vi "Pack PII Error_1SDI_v00.vi"(8 "PII+Error HD C":T1, 9 "PII+Error HD B":T1, 10 "PII+Error HD A":T1, 11 "PII+Error EPR BS":T8) -> (0 "Theta":T5, 1 "Thresholds":cluster{"Lock":T7, "Re-Scan":T7}, 3 "Error packed":T6={"Pre-Offset"={"Pre-Offset 1"=2, "Pre-Offset 2"=0, "Pre-Offset 3"=0, "Pre-Offset 4"=0, "Pre-Offset 5"=2, "Pre-Offset 6"=0, "Pre-Offset 7"=2}, "Post-Offset "={"Offset 1"=0, "Offset 2"=0, "Offset 3"=0, "Offset 4"=0, "Offset 5"=0, "Offset 6"=0, "Offset 7"=0}, "Gains"={"Gain 1"=0, "Gain 2"=0, "Gain 3"=0, "Gain 4"=0, "Gain 5"=0, "Gain 6"=0, "Gain 7"=0}, "Bit Shifts"={"Bit Shift 1"=0, "Bit Shift 2"=300, "Bit Shift 3"=0, "Bit Shift 4"=0, "Bit Shift 5"=0, "Bit Shift 6"=0, "Bit Shift 7"=0}})   [LabVIEW 2013]
doc: "Packages individual values related to error signal scaling from the user interface into data structures compatible with FPGA_Cavities.VI\n(very messy, could use a tidy)."
uses:
  Strict Type Defs/1SDI Errors I16.ctl
  Strict Type Defs/Error Scale 1SDI.ctl
  Strict Type Defs/PII and Error Graph.ctl
  Strict Type Defs/Errors Converted Graph.ctl
  Strict Type Defs/PII individual.ctl
  Strict Type Defs/PII and Error Graph HD.ctl
  Strict Type Defs/Errors Converted Graph HD.ctl
  Strict Type Defs/Lock Thresh 1SDI.ctl
  Strict Type Defs/Theta graph.ctl
panel:
  in  "Bit Shifts":T4
  in  "Theta typedef":T5
  in  "Error scale graph type":T6={"Pre-Offset"={"Pre-Offset 1"=2, "Pre-Offset 2"=0, "Pre-Offset 3"=0, "Pre-Offset 4"=0, "Pre-Offset 5"=2, "Pre-Offset 6"=0, "Pre-Offset 7"=2}, "Post-Offset "={"Offset 1"=0, "Offset 2"=300, "Offset 3"=0, "Offset 4"=0, "Offset 5"=0, "Offset 6"=0, "Offset 7"=0}, "Gains"={"Gain 1"=0, "Gain 2"=300, "Gain 3"=0, "Gain 4"=0, "Gain 5"=0, "Gain 6"=0, "Gain 7"=0}, "Bit Shifts"={"Bit Shift 1"=0, "Bit Shift 2"=300, "Bit Shift 3"=0, "Bit Shift 4"=0, "Bit Shift 5"=0, "Bit Shift 6"=0, "Bit Shift 7"=0}}
  in  "Thresholds type def":cluster{"Lock":T7, "Re-Scan":T7}
  in  "Re-Scan Thresh":T7
  in  "Lock Thresh":T7
  in  "Pre Offset":T4
  in  "Offset":T4
  in  "Gains":T4
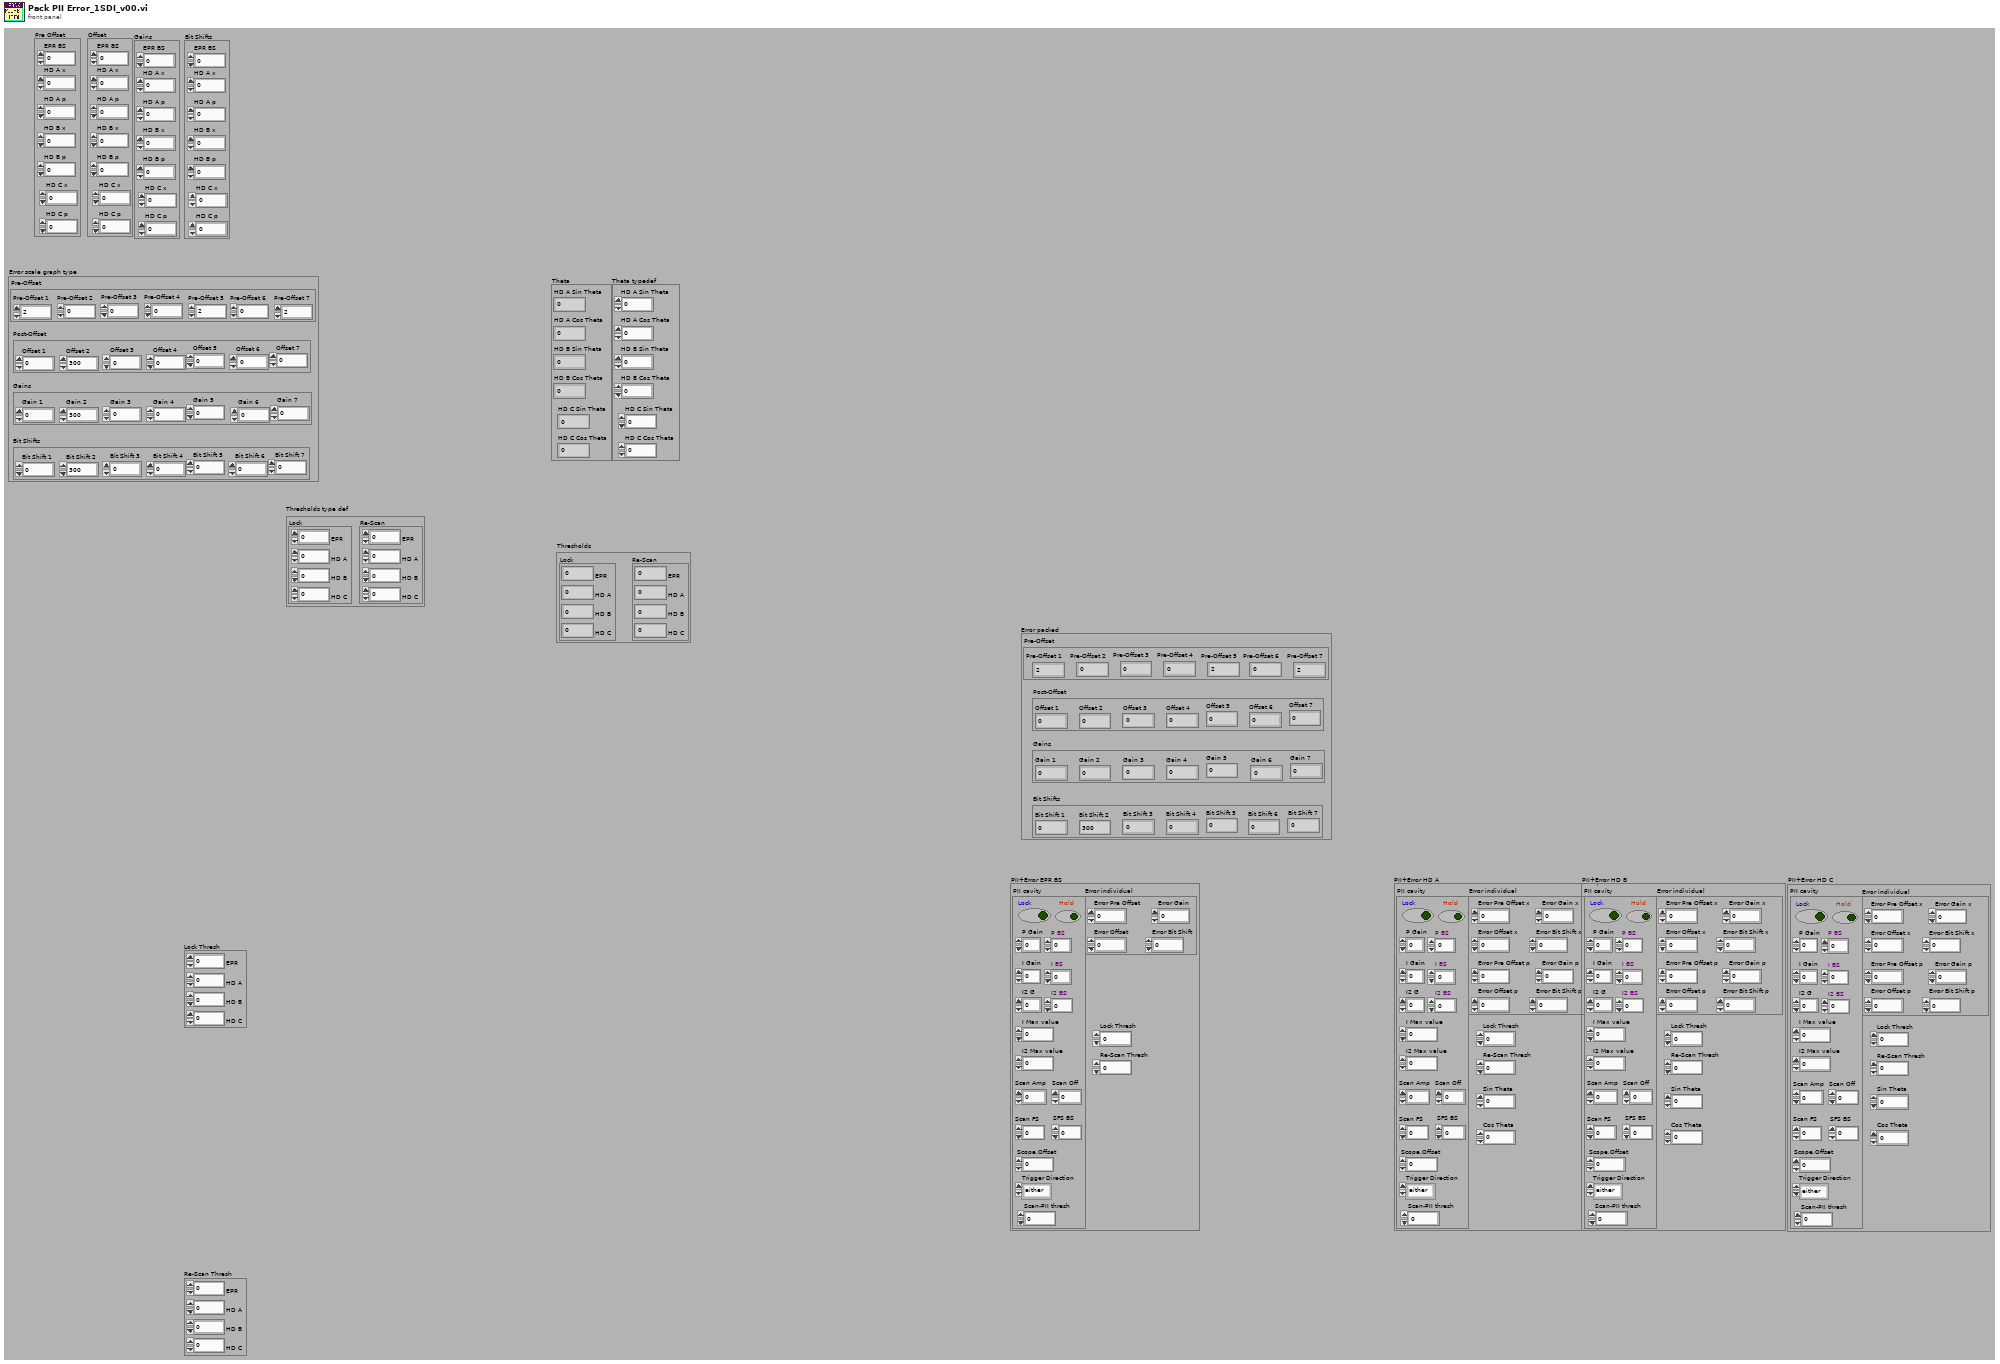
[diagram p1: front panel]
types:
  T1 = typedef "PII and Error Graph HD.ctl" = cluster{"Error individual":T2, "PII cavity":T3, "Lock Thresh":i16, "Re-Scan Thresh":i16, "Sin Theta":i32, "Cos Theta":i32}
  T2 = typedef "Errors Converted Graph HD.ctl" = cluster{"Error Pre Offset x":i16, "Error Offset x":i16, "Error Gain x":i16, "Error Bit Shift x":i16, "Error Pre Offset p":i16, "Error Offset p":i16, "Error Gain p":i16, "Error Bit Shift p":i16}
  T3 = typedef "PII individual.ctl" = cluster{"Lock":bool, "Hold":bool, "P Gain":i32, "P BS":i16, "I Gain":i32, "I BS":i16, "I2 G":i32, "I2 BS":i16, "Scan Amp":i16, "Scan Off":i16, "Scan FS":u16, "SFS BS":i16, "I Max value":i32, "I2 Max value":i32, "Scope.Offset":i16, "Trigger Direction":enum8{"either", "minus-plus", "plus-minus"}, "Scan-PII thresh":i16}
  T4 = typedef "1SDI Errors I16.ctl" = cluster{"EPR BS":i16, "HD A x":i16, "HD A p":i16, "HD B x":i16, "HD B p":i16, "HD C p":i16, "HD C x":i16}
  T5 = typedef "Theta graph.ctl" = cluster{"HD A Sin Theta":i32, "HD A Cos Theta":i32, "HD B Sin Theta":i32, "HD B Cos Theta":i32, "HD C Sin Theta":i32, "HD C Cos Theta":i32}
  T6 = typedef "Error Scale 1SDI.ctl" = cluster{"Pre-Offset":cluster{"Pre-Offset 1":i16, "Pre-Offset 2":i16, "Pre-Offset 3":i16, "Pre-Offset 4":i16, "Pre-Offset 5":i16, "Pre-Offset 6":i16, "Pre-Offset 7":i16}, "Post-Offset ":cluster{"Offset 1":i16, "Offset 2":i16, "Offset 3":i16, "Offset 4":i16, "Offset 5":i16, "Offset 6":i16, "Offset 7":i16}, "Gains":cluster{"Gain 1":i16, "Gain 2":i16, "Gain 3":i16, "Gain 4":i16, "Gain 5":i16, "Gain 6":i16, "Gain 7":i16}, "Bit Shifts":cluster{"Bit Shift 1":i16, "Bit Shift 2":i16, "Bit Shift 3":i16, "Bit Shift 4":i16, "Bit Shift 5":i16, "Bit Shift 6":i16, "Bit Shift 7":i16}}
  T7 = typedef "Lock Thresh 1SDI.ctl" = cluster{"EPR":i16, "HD A":i16, "HD B":i16, "HD C":i16}
  T8 = typedef "PII and Error Graph.ctl" = cluster{"Error individual":T9, "PII cavity":T3, "Lock Thresh":i16, "Re-Scan Thresh":i16}
  T9 = typedef "Errors Converted Graph.ctl" = cluster{"Error Pre Offset":i16, "Error Offset":i16, "Error Gain":i16, "Error Bit Shift":i16}
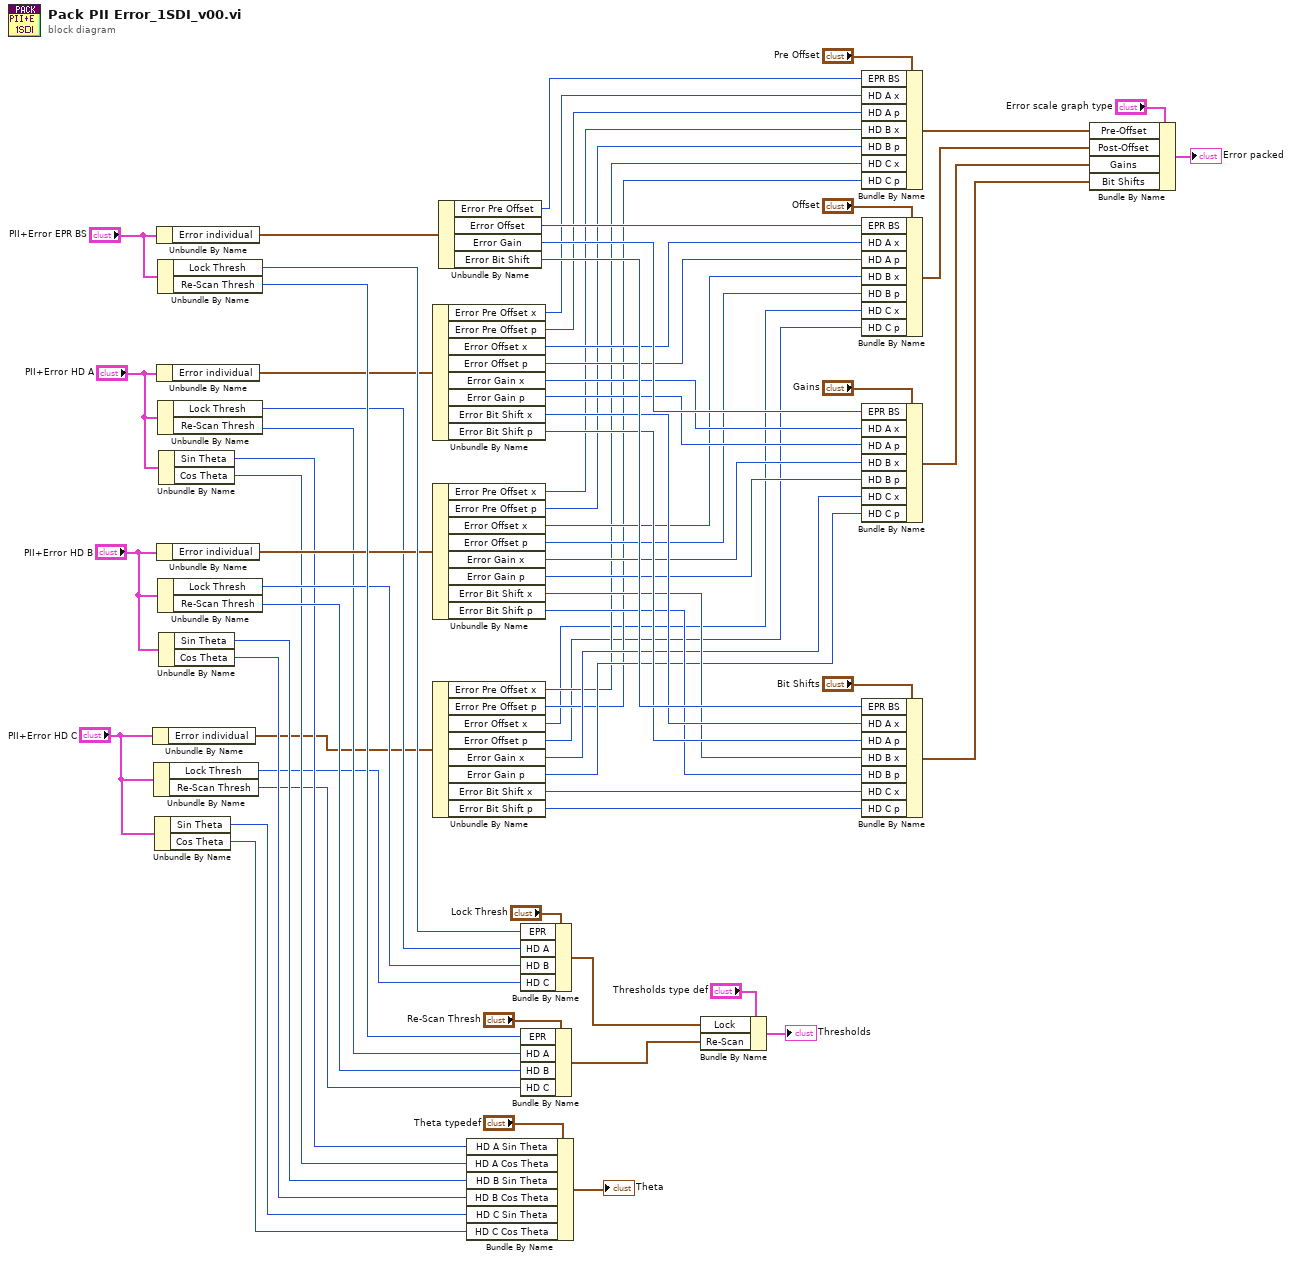
[diagram p0: block diagram]
diagram:
  n1 = Unbundle By Name("PII+Error HD C") -> ("Error individual"=w13:T2)
  n2 = Unbundle By Name("PII+Error HD C") -> ("Lock Thresh"=w12:i16, "Re-Scan Thresh"=w11:i16)
  n3 = Unbundle By Name("PII+Error HD C") -> ("Sin Theta"=w10:i32, "Cos Theta"=w9:i32)
  n4 = Unbundle By Name("PII+Error EPR BS") -> ("Error individual"=w67:T9)
  n5 = Unbundle By Name("PII+Error HD A") -> ("Error individual"=w46:T2)
  n6 = Unbundle By Name("PII+Error HD B") -> ("Error individual"=w37:T2)
  n7 = Unbundle By Name("PII+Error EPR BS") -> ("Lock Thresh"=w59:i16, "Re-Scan Thresh"=w57:i16)
  n8 = Unbundle By Name("PII+Error HD A") -> ("Lock Thresh"=w28:i16, "Re-Scan Thresh"=w26:i16)
  n9 = Unbundle By Name("PII+Error HD B") -> ("Lock Thresh"=w27:i16, "Re-Scan Thresh"=w25:i16)
  n10 = Unbundle By Name("PII+Error HD A") -> ("Sin Theta"=w23:i32, "Cos Theta"=w22:i32)
  n11 = Unbundle By Name("PII+Error HD B") -> ("Sin Theta"=w20:i32, "Cos Theta"=w19:i32)
  n12 = Unbundle By Name(w46) -> ("Error Pre Offset x"=w45:i16, "Error Pre Offset p"=w44:i16, "Error Offset x"=w43:i16, "Error Offset p"=w42:i16, "Error Gain x"=w41:i16, "Error Gain p"=w40:i16, "Error Bit Shift x"=w39:i16, "Error Bit Shift p"=w38:i16)
  n13 = Unbundle By Name(w37) -> ("Error Pre Offset x"=w29:i16, "Error Pre Offset p"=w30:i16, "Error Offset x"=w31:i16, "Error Offset p"=w32:i16, "Error Gain x"=w33:i16, "Error Gain p"=w34:i16, "Error Bit Shift x"=w35:i16, "Error Bit Shift p"=w36:i16)
  n14 = Unbundle By Name(w13) -> ("Error Pre Offset x"=w4:i16, "Error Pre Offset p"=w3:i16, "Error Offset x"=w2:i16, "Error Offset p"=w1:i16, "Error Gain x"=w5:i16, "Error Gain p"=w6:i16, "Error Bit Shift x"=w8:i16, "Error Bit Shift p"=w7:i16)
  n15 = Unbundle By Name(w67) -> ("Error Pre Offset"=w66:i16, "Error Offset"=w65:i16, "Error Gain"=w64:i16, "Error Bit Shift"=w47:i16)
  n16 = Bundle By Name(cluster="Theta typedef", "HD A Sin Theta"=w23, "HD A Cos Theta"=w22, "HD B Sin Theta"=w20, "HD B Cos Theta"=w19, "HD C Sin Theta"=w10, "HD C Cos Theta"=w9) -> (→"Theta":T5)
  n17 = Bundle By Name(cluster="Lock Thresh", "EPR"=w59, "HD A"=w28, "HD B"=w27, "HD C"=w12) -> (w55:T7)
  n18 = Bundle By Name(cluster="Re-Scan Thresh", "EPR"=w57, "HD A"=w26, "HD B"=w25, "HD C"=w11) -> (w54:T7)
  n19 = Bundle By Name(cluster="Thresholds type def", "Lock"=w55, "Re-Scan"=w54) -> (→"Thresholds":cluster{"Lock":T7, "Re-Scan":T7})
  n20 = Bundle By Name(cluster="Pre Offset", "EPR BS"=w66, "HD A x"=w45, "HD A p"=w44, "HD B x"=w29, "HD B p"=w30, "HD C x"=w4, "HD C p"=w3) -> (w18:T4)
  n21 = Bundle By Name(cluster="Offset", "EPR BS"=w65, "HD A x"=w43, "HD A p"=w42, "HD B x"=w31, "HD B p"=w32, "HD C x"=w2, "HD C p"=w1) -> (w17:T4)
  n22 = Bundle By Name(cluster="Gains", "EPR BS"=w64, "HD A x"=w41, "HD A p"=w40, "HD B x"=w33, "HD B p"=w34, "HD C x"=w5, "HD C p"=w6) -> (w16:T4)
  n23 = Bundle By Name(cluster="Bit Shifts", "EPR BS"=w47, "HD A x"=w39, "HD A p"=w38, "HD B x"=w35, "HD B p"=w36, "HD C x"=w8, "HD C p"=w7) -> (w15:T4)
  n24 = Bundle By Name(cluster="Error scale graph type", "Pre-Offset"=w18, "Post-Offset"=w17, "Gains"=w16, "Bit Shifts"=w15) -> (→"Error packed":T6)
